vi "Vision Server Restart ADB.vi"(1 "error in":errorcluster, 2 "Vision Server":T1) -> (0 "error out":errorcluster)   [LabVIEW 2016]
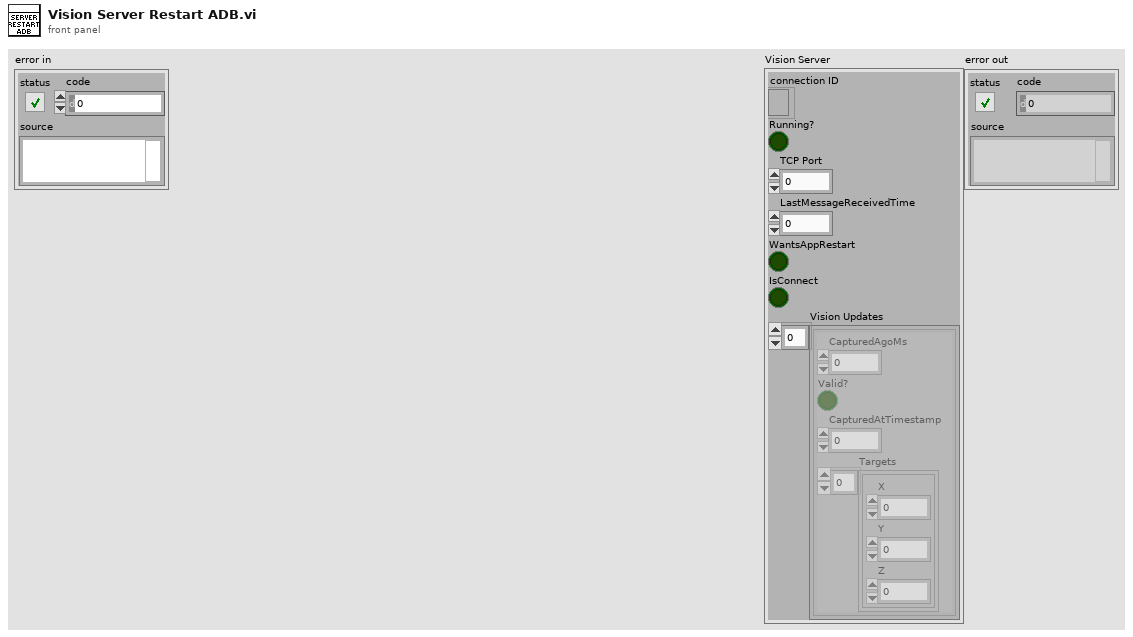
[diagram p1: front panel]
types:
  T1 = cluster{"connection ID":refnum<k5>, "Running?":bool, "TCP Port":u16, "LastMessageReceivedTime":dbl, "WantsAppRestart":bool, "IsConnect":bool, "Vision Updates":cluster{"CapturedAgoMs":i32, "Valid?":bool, "CapturedAtTimestamp":dbl, "Targets":cluster{"X":dbl, "Y":dbl, "Z":dbl}[]}[]}
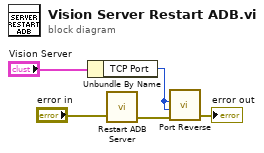
[diagram p0: block diagram]
diagram:
  n1 = Unbundle By Name("Vision Server") -> ("TCP Port"=w3:u16)
  n2 = call "Restart ADB Server.vi"("error in"="error in") -> ("error out"=w2:errorcluster)  [unwired: 1 in, 2 out]
  n3 = call "Port Reverse.vi"("error in"=w2, "local TCP port"=w3, "remote TCP port"=w3) -> ("error out"=→"error out":errorcluster)  [unwired: 1 in, 2 out]
